vi "TestStringConcatWithHex.vi"() -> ()   [LabVIEW 2012]
panel:
  out "Data Return":string[](array[string])
  out "Command Out":string
  out "What to Do":string="Interpret this response from MCS"
  out "concatenated string":string
  in  "HexString":string="\u0000\u0000CM"
  in  "String":string="MCS_NCAR_"
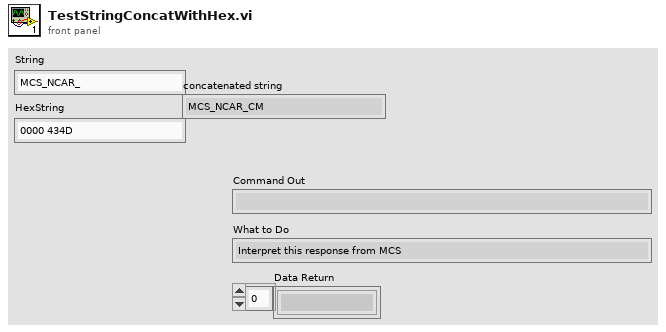
[diagram p1: front panel]
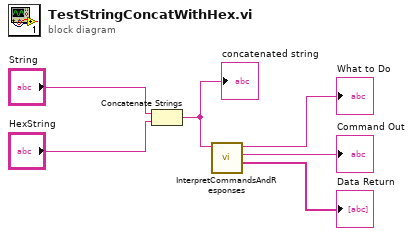
[diagram p0: block diagram]
diagram:
  n1 = Concatenate Strings("String", "HexString") -> (w4:string)
  "concatenated string" <- w4
  n2 = call "InterpretCommandsAndResponses.vi"("Input Command"=w4) -> ("Data Return"=→"Data Return":string[], "Command Out"=→"Command Out":string, "What to Do"=→"What to Do":string)  [unwired: 7 in, 1 out]
